vi "testUnflattenMassFromXML.vi"() -> ()   [LabVIEW 2012, in "UnitsAndXML.lvlib"]
uses:
  <userlib>/Common/UnitsAndXML/UnitsAndXML.lvlib
  <userlib>/Common/UnitsAndXML/FlattenItemWithUnitToXML/FlattenMassToXML/MassUnit.ctl
  <userlib>/Common/UnitsAndXML/UnflattenItemWithUnitFromXML/UnflattenMassFromXML/typeMethods/unflattenMassFromXML_Array.vi
  <userlib>/Common/UnitsAndXML/UnflattenItemWithUnitFromXML/UnflattenMassFromXML/typeMethods/unflattenMassFromXML_Scalar.vi
panel:
  out "error out":errorcluster
  out "mass":dbl[unit][](array[numeric])
  out "mass":dbl[unit]
  in  "massUnitInXML":T1
  in  "xmlStringArray":string="<mass>15</mass>\r\n<mass>30</mass>\r\n<mass>45</mass>\r\n<mass>60</mass>"
  in  "xmlStringScalar":string="<mass>15</mass>"
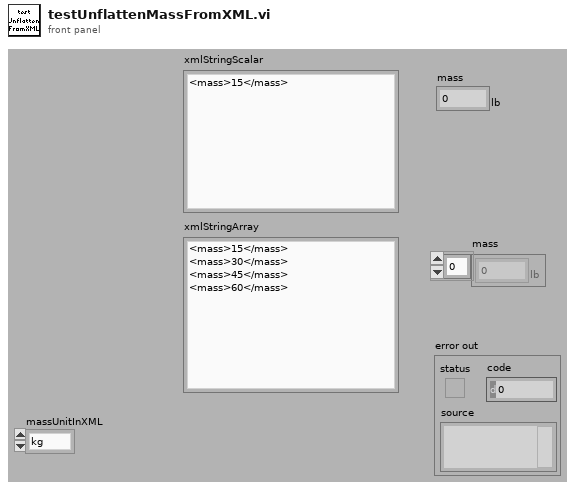
[diagram p1: front panel]
types:
  T1 = typedef "UnitsAndXML.lvlib/MassUnit.ctl" = enum16{"kg", "CM", "dr", "gr", "t", "oz", "lb", "slug", "stone", "Ton", "ton", "u"}
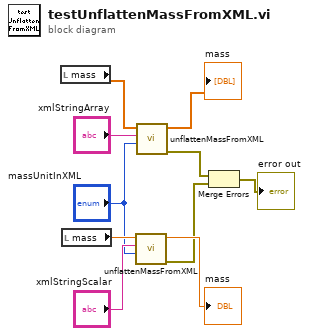
[diagram p0: block diagram]
diagram:
  n1 = local read "mass"() -> (w3:dbl[unit][])
  n2 = local read "mass"() -> (w9:dbl[unit])
  n3 = call-poly <userlib>:"unflattenMassFromXML.vi"("massUnitInXML"="massUnitInXML", "xmlString"="xmlStringScalar", "massForType"=w9) -> ("error out"=w5:errorcluster, "mass"=→"mass":dbl[unit])  [unwired: 7 in]
  n4 = call-poly <userlib>:"unflattenMassFromXML.vi"("massUnitInXML"="massUnitInXML", "xmlString"="xmlStringArray", "massForType"=w3) -> ("error out"=w6:errorcluster, "mass"=→"mass":dbl[unit][])  [unwired: 7 in]
  n5 = Merge Errors(w6, w5) -> (→"error out":errorcluster)
